vi "TrackFrequencies.vi"(8 "freq_array":dbl[][](array[numeric]), 9 "sig_Y":dbl[](array[numeric]), 10 "sig_X":dbl[](array[numeric]), 11 "freqs":dbl[](array[numeric])) -> (1 "new_freq_array":dbl[][](array[numeric]))   [LabVIEW 2015]
uses:
  <vilib>/imath/engines/lvmath2/RunTimeEngine/BitwiseOperatorToken/NIMS_Bitwise_Operator_And.vi
  <instcachedir>/0/NIMS_Bitwise_Operator_And_B0AE5782C74E9A449AB5F55AFA3AE827.lvgen/NIMS_Bitwise_Operator_And_B0AE5782C74E9A449AB5F55AFA3AE827_001.vi
  <vilib>/imath/engines/lvmath2/RunTimeEngine/VariableToken/Support/NIMS_Vector Boolean Index to I32 Index.vi
  <vilib>/imath/engines/lvmath2/RunTimeEngine/IndexRead/NIMS V(V).vi
  <instcachedir>/0/NIMS V(V)_298D9CB7BFEB42B8BC8D9C3C28AE8C70.lvgen/NIMS V(V)_298D9CB7BFEB42B8BC8D9C3C28AE8C70_000.vi
  <vilib>/imath/engines/lvmath2/RunTimeEngine/ErrorHandling/NIMS_Create Error From Enums.vi
  <vilib>/imath/engines/lvmath2/RunTimeEngine/NodeEndStatement/NIMS_NodeEndStatement_Output.vi
  <instcachedir>/0/NIMS_NodeEndStatement_Output_53EC0D466D134D7ABD903AC30B43404B.lvgen/NIMS_NodeEndStatement_Output_53EC0D466D134D7ABD903AC30B43404B_005.vi
  <vilib>/imath/engines/lvmath2/RunTimeEngine/ErrorHandling/NIMS_Finalize Error.vi
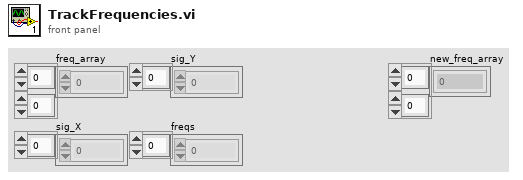
[diagram p1: front panel]
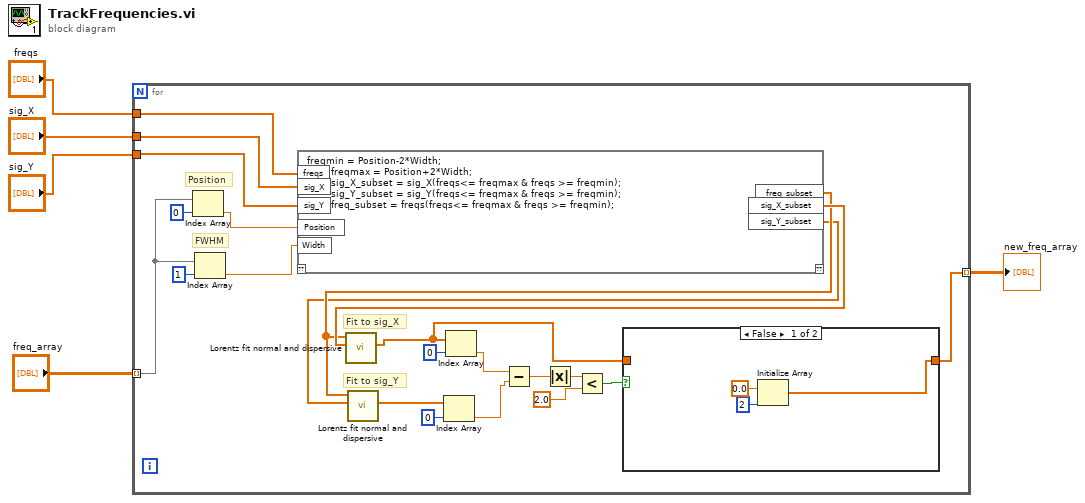
[diagram p0: block diagram]
diagram:
  n1 = for {
    tunnel: "freq_array" -> [w27] mode=indexing
    tunnel: "sig_Y" -> [w20]
    tunnel: "sig_X" -> [w21]
    tunnel: "freqs" -> [w22]
    tunnel: [w6] -> w1 mode=indexing
    # "Fit to sig_Y"
    # "Fit to sig_X"
    # "FWHM"
    # "Position"
    n2 = Index Array(array=w27, index=0) -> (element=w24:dbl)
    n3 = Index Array(array=w27, index=1) -> (element=w23:dbl)
    n4 = mathscript code="freqmin = Position-2*Width;\n        freqmax = Position+2*Width;\n        sig_X_subset = sig_X(freqs<= freqmax & freqs >= freqmin);\n        sig_Y_subset = sig_Y(freqs<= freqmax & freqs >= freqmin);\n        freq_subset = freqs(freqs<= freqmax & freqs >= freqmin);"("freqs"=w22, "sig_X"=w21, "sig_Y"=w20, "Position"=w24, "Width"=w23) -> ("freq_subset"=w18:dbl[], "sig_X_subset"=w19:dbl[], "sig_Y_subset"=w17:dbl[])  [unwired: 1 in, 1 out]
    n5 = call "Lorentz fit normal and dispersive.vi"("Y subset"=w19, "X subset"=w18) -> ("Position/FWHM"=w7:dbl[])  [unwired: 5 in, 4 out]
    n6 = call "Lorentz fit normal and dispersive.vi"("Y subset"=w17, "X subset"=w18) -> ("Position/FWHM"=w14:dbl[])  [unwired: 5 in, 4 out]
    n7 = Index Array(array=w14, index=0) -> (element=w12:dbl)
    n8 = Index Array(array=w7, index=0) -> (element=w13:dbl)
    n9 = Subtract(x=w13, y=w12) -> (x-y=w11:dbl)
    n10 = Absolute Value(x=w11) -> (abs(x)=w10:dbl)
    n11 = Less?(x=w10, y=2.0) -> (x < y?=w8:bool)
    n12 = case shown="False" w8 {
      tunnel: w7 -> [_ w31]
      tunnel: [w28 w31] -> w6
      frame False {
        n13 = Initialize Array(0.0 ("element"), 2 ("dimension size")) -> (w28:dbl[])
      }
      frame True {
      }
    }
  }
  "new_freq_array" <- w1
